vi "Read Analog Variable Setups from Ini.vi"(0 "error in (no error)":errorcluster, 1 "Path":path, 7 "Enum with Variable List":variant, 12 "Section(\"Default\")":string="Default") -> (4 "error out":errorcluster, 6 "Found out":bool[](array[boolean]), 8 "Analog User settigns":T1[](array[typedef]) {"Scaling"."Offset" format="%.5f"; "Scaling"."Gain" format="%.5f"; "Limits and responces"."Limits"."H" format="%.3f"; "Limits and responces"."Limits"."L" format="%.3f"; "Limits and responces"."Limits"."HH" format="%.3f"; "Limits and responces"."Limits"."LL" format="%.3f"})   [LabVIEW 2011]
uses:
  User Setting Analog Channel Bg.ctl
  Scaling.ctl
  Alarm Setup Analog.ctl
  Alarm Responce.ctl
  Action List.ctl
  Limits.ctl
  <vilib>/Utility/VariantDataType/GetNumericInfo.vi
  <vilib>/Utility/libraryn.llb/Check if File or Folder Exists.vi
  <vilib>/Utility/config.llb/NI_LVConfig.lvlib
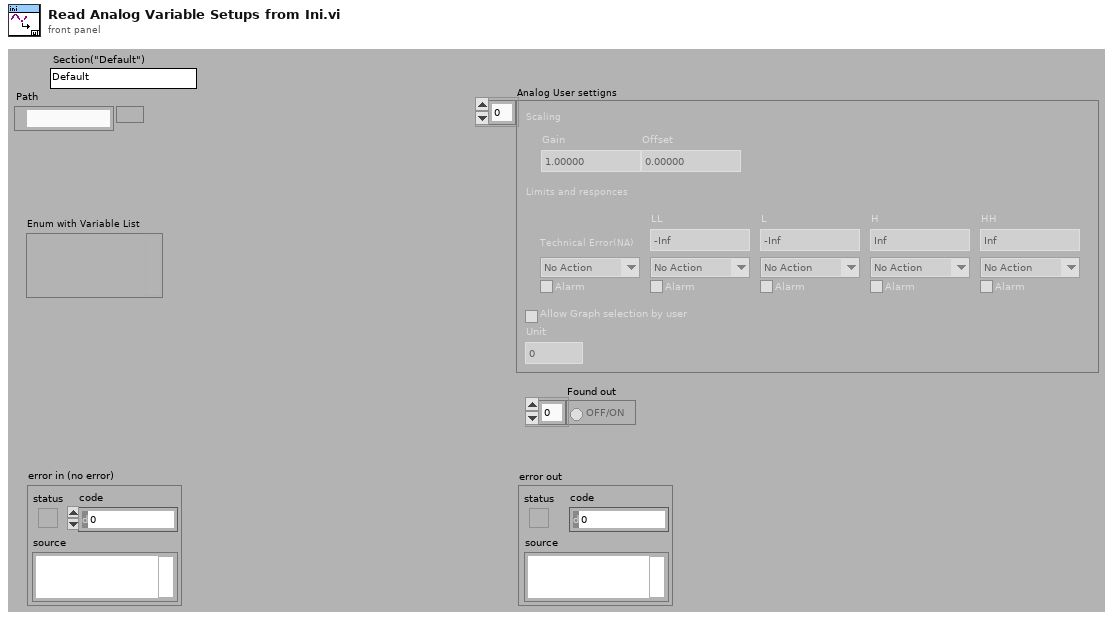
[diagram p1: front panel]
types:
  T1 = typedef "User Setting Analog Channel Bg.ctl" = cluster{"Scaling":T2, "Limits and responces":T3, "Allow Graph selection by user":bool, "Unit":u16}
  T2 = typedef "Scaling.ctl" = cluster{"Gain":dbl, "Offset":dbl}
  T3 = typedef "Alarm Setup Analog.ctl" = cluster{"Technical Error(NA)":T4, "LL":T4, "L":T4, "H":T4, "HH":T4, "Limits":T6}
  T4 = typedef "Alarm Responce.ctl" = cluster{"Action":T5, "Alarm":bool}
  T5 = typedef "Action List.ctl" = enum16{"No Action", "Stop Motor", "Turn Off HV"}
  T6 = typedef "Limits.ctl" = cluster{"LL":dbl, "L":dbl, "H":dbl, "HH":dbl}
  T7 = typedef "NI_LVConfig.lvlib/Config Data RefNum.ctl" = refnum<k1>
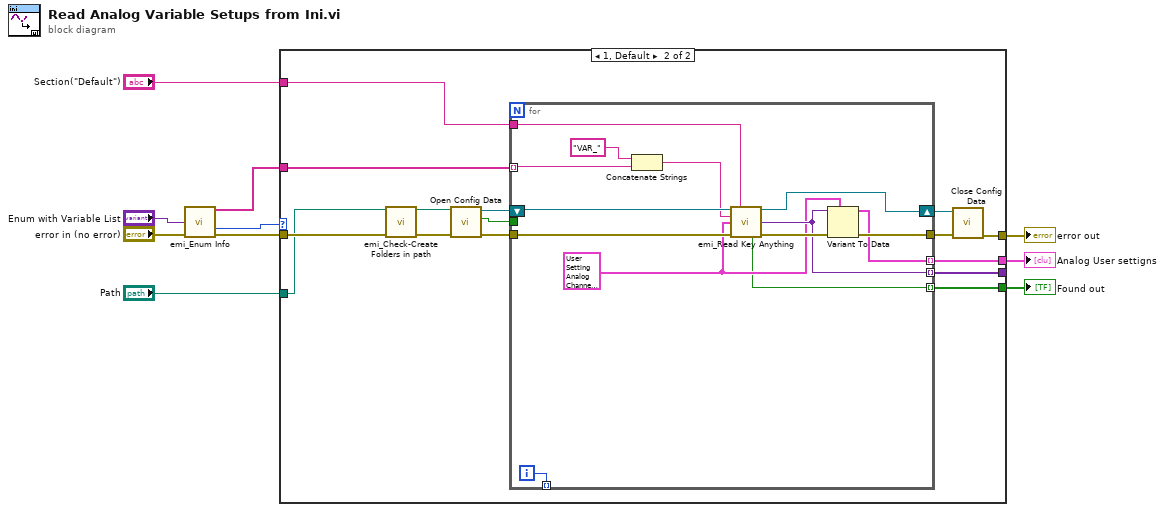
[diagram p0: block diagram]
diagram:
  n1 = call "emi_Enum Info.vi"("Enum"="Enum with Variable List", "error in (no error)"="error in (no error)") -> ("Text Elements"=w6:string[], "Numb Elements"=w7:i32, "error out"=w4:errorcluster)  [unwired: 10 in, 1 out]
  n2 = case shown="1, Default" w7 {
    tunnel: w6 -> [_ w24]
    tunnel: w4 -> [w11 w16]
    tunnel: [w11 w21] -> w10
    tunnel: [_ w20] -> w9
    tunnel: "Path" -> [_ w15]
    tunnel: "Section(\"Default\")" -> [_ w17]
    tunnel: [_ w14] -> _
    tunnel: [_ w12] -> w1
    frame 0 {
    }
    frame 1, Default {
      n3 = call "emi_Check-Create Folders in path.vi"("Path including file"=w15, "error in (no error)"=w16) -> ("Path out"=w18:path, "error out"=w19:errorcluster)  [unwired: 11 in, 1 out]
      n4 = call <vilib>:"Open Config Data.vi"("error in (no error)"=w19, "configuration file path"=w18) -> ("error out"=w26:errorcluster, "file created?"=w13:bool, "refnum"=w25:T7)  [unwired: 7 in]
      n5 = for {
        tunnel: w24 -> [w31] mode=indexing
        tunnel: w26 -> [w39]
        tunnel: w17 -> [w38]
        tunnel: [w34] -> w23
        shift-right: [w33] -> w22
        shift-left: w25 -> [w37]
        tunnel: [w32] -> w20 mode=indexing
        tunnel: [w30] -> _ mode=indexing
        tunnel: [w29] -> w14 mode=indexing
        tunnel: w13 -> [_]
        tunnel: [w27] -> w12 mode=indexing
        i -> [w30]
        w28 = T1 {"Scaling"={"Gain"=1.0, "Offset"=0.0}, "Limits and responces"={"Technical Error(NA)"={"Action"=enum."No Action", "Alarm"=FALSE}, "LL"={"Action"=enum."No Action", "Alarm"=FALSE}, "L"={"Action"=enum."No Action", "Alarm"=FALSE}, "H"={"Action"=enum."No Action", "Alarm"=FALSE}, "HH"={"Action"=enum."No Action", "Alarm"=FALSE}, "Limits"={"LL"=-inf, "L"=-inf, "H"=inf, "HH"=inf}}, "Allow Graph selection by user"=FALSE, "Unit"=0} ("User Selectable")
        n6 = Concatenate Strings("VAR_" ("string"), w31) -> (w35:string)
        n7 = call "emi_Read Key Anything.vi"("Ini file refnum"=w37, "Section(Default)"=w38, "Name"=w35, "Anything"=w28, "error in (no error)"=w39) -> ("Ini file refnum out"=w33:T7, "Anything Out"=w29:variant, "Found"=w27:bool, "error out"=w36:errorcluster)  [unwired: 7 in]
        n8 = Variant To Data(error in=w36, type=w28, Variant=w29) -> (data=w32:T1, error out=w34:errorcluster)
      }
      n9 = call <vilib>:"Close Config Data.vi"("error in (no error)"=w23, "refnum"=w22) -> ("error out"=w21:errorcluster)  [unwired: 8 in, 1 out]
    }
  }
  "Analog User settigns" <- w9
  "error out" <- w10
  "Found out" <- w1
